vi "sub_ofdm_cp_removed.vi"(9 "CP length":i32=64, 11 "time ofdm symbol":cdb[](array[numeric])) -> (3 "cp removed ofdm symbol":cdb[](array[numeric]))   [LabVIEW 2014]
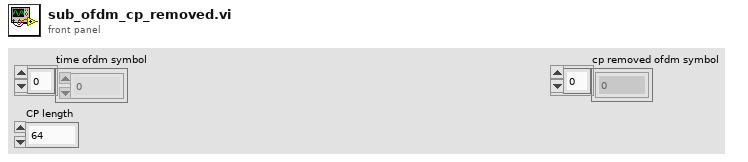
[diagram p1: front panel]
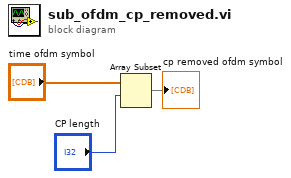
[diagram p0: block diagram]
diagram:
  n1 = Array Subset(array="time ofdm symbol", index="CP length") -> (→"cp removed ofdm symbol":cdb[])  [unwired: 1 in]
